vi "LWXPS_EventExtendedConfigurationActionGet.vi"(0 "XPS Reference IN":refnum<k24>, 11 "LabVIEW error IN":errorcluster) -> (4 "XPS Reference OUT":refnum<k24>, 6 "Returned error code":i32, 8 "Action Configuration":string, 10 "XPS Error String":string, 15 "LabVIEW error OUT":errorcluster)   [LabVIEW 2014]
uses:
  D:/XPSQ8_LabView_Library/Development/Source/Dll/Newport.XPS.CommandInterface.dll
  Dll/Newport.XPS.CommandInterface.dll
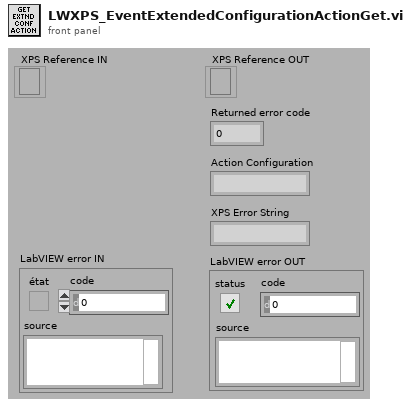
[diagram p1: front panel]
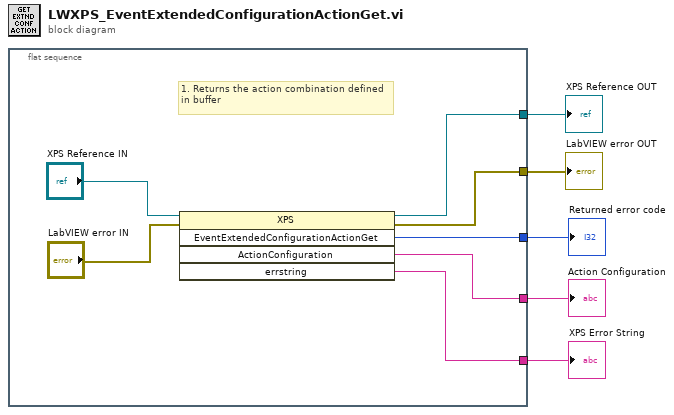
[diagram p0: block diagram]
diagram:
  n1 = flat-sequence {
    tunnel: [w6] -> w2
    tunnel: [w10] -> w1
    tunnel: [w9] -> w5
    tunnel: [w8] -> w4
    tunnel: [w7] -> w3
    frame #0 {
      # "1. Returns the action combination defined in buffer"
      n2 = invoke class="XPS" method="EventExtendedConfigurationActionGet"(reference="XPS Reference IN", error in="LabVIEW error IN") -> (reference out=w9:refnum<k24>, error out=w8:errorcluster, "EventExtendedConfigurationActionGet"=w7:i32, "ActionConfiguration"=w6:string, "errstring"=w10:string)  [unwired: 3 in]
    }
  }
  "XPS Reference OUT" <- w5
  "LabVIEW error OUT" <- w4
  "Returned error code" <- w3
  "Action Configuration" <- w2
  "XPS Error String" <- w1
